vi "Calculate new Timeout.vi"(6 "Start Time":u32, 7 "Total Timeout":i32, 8 "Error In":errorcluster) -> (0 "Error Out":errorcluster, 5 "remaining Timeout":i32)   [LabVIEW 2011, in "Tinkerforge.lvlib" / "IP Connection.lvclass"]
doc: "This VI calculates the remaining timeout."
uses:
  IP Connection.lvclass
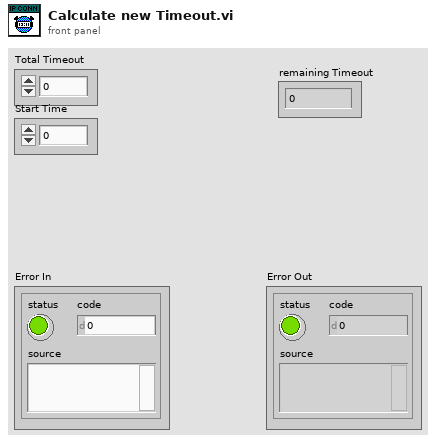
[diagram p1: front panel]
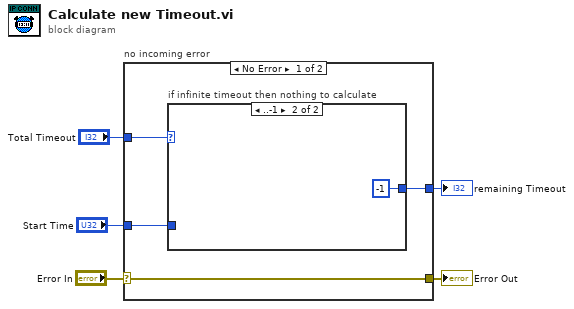
[diagram p0: block diagram]
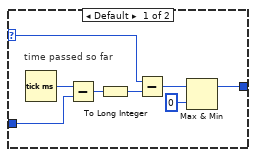
[diagram p2: hidden frame]
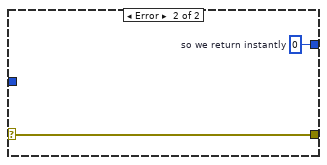
[diagram p3: hidden frame]
diagram:
  n1 = case "no incoming error" shown="No Error" "Error In" {
    selector: "Error In" -> [w9 w20]
    tunnel: [w9 w20] -> w4
    tunnel: "Total Timeout" -> [w8 _]
    tunnel: "Start Time" -> [w7 _]
    tunnel: [w6 w19] -> w1
    frame No Error {
      n2 = case "if infinite timeout then nothing to calculate" shown="..-1" w8 {
        selector: w8 -> [w14 _]
        tunnel: w7 -> [w16 _]
        tunnel: [w10 -1] -> w6
        frame Default {
          # "time passed so far"
          n3 = Tick Count (ms)() -> (millisecond timer value=w17:u32)
          n4 = Subtract(x=w17, y=w16) -> (x-y=w15:u32)
          n5 = To Long Integer(number=w15) -> (32bit integer=w13:i32)
          n6 = Subtract(x=w14, y=w13) -> (x-y=w12:i32)
          n7 = Max & Min(x=w12, y=0) -> (max(x,y)=w10:i32)  [unwired: 1 out]
        }
        frame ..-1 {
        }
      }
    }
    frame Error {
      w19 = 0  # so we return instantly
    }
  }
  "Error Out" <- w4
  "remaining Timeout" <- w1
